vi "AWG Set and Arm.vi"(8 "error in (no error)":errorcluster, 10 "T [s] (1ms)":dbl=0.001, 11 "awg session in":T1) -> (0 "error out":errorcluster, 3 "awg session out":T1)   [LabVIEW 2018, in "AWG.lvlib"]
doc: "AWG wrapper: This sets the AWG to desired frequency and arms it. No pulses are generated here. Waiting for trigger!"
uses:
  AWG.lvlib
  AWG Session.ctl
  AWG Type.ctl
  Agilent 33XXX Series/Agilent 33XXX Series.lvlib
  AFG3000/Tektronix AFG 3000 Series.lvlib
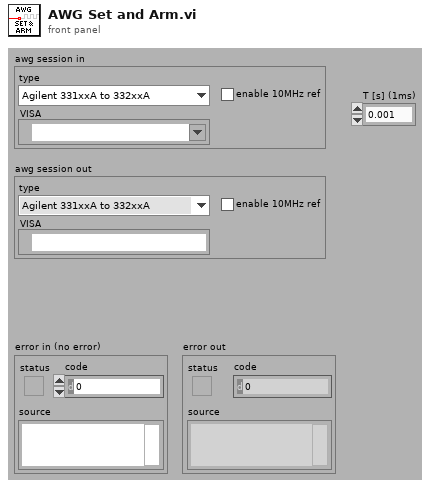
[diagram p1: front panel]
types:
  T1 = typedef "AWG.lvlib/AWG Session.ctl" = cluster{"type":T2, "VISA":refnum<visa-resource-name>, "enable 10MHz ref":bool}
  T2 = typedef "AWG.lvlib/AWG Type.ctl" = enum16{"Agilent 331xxA to 332xxA", "Agilent 335xxA to 336xxA", "Tektronix AFG3101C", "dummy"}
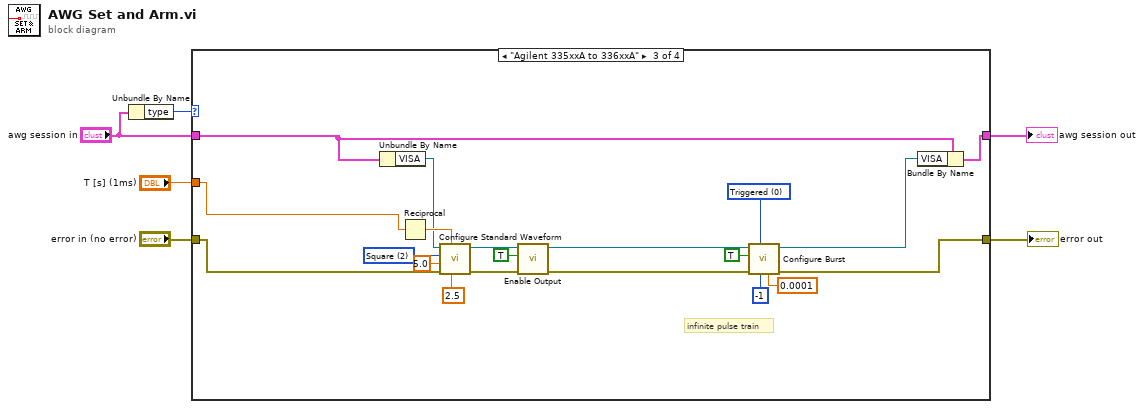
[diagram p0: block diagram]
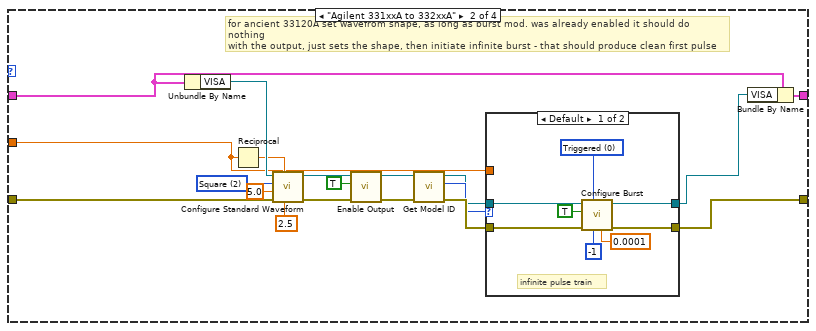
[diagram p3: hidden frame]
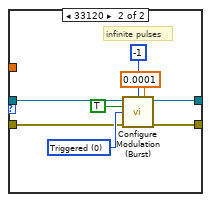
[diagram p4: hidden frame]
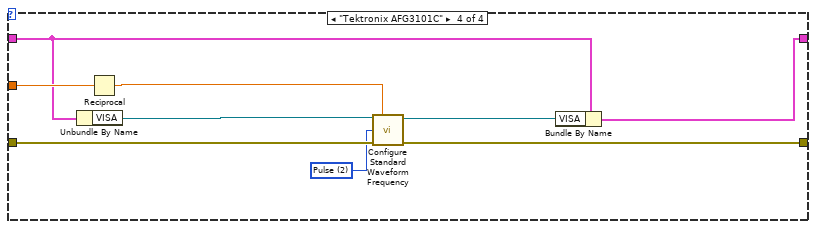
[diagram p5: hidden frame]
diagram:
  n1 = Unbundle By Name("awg session in") -> ("type"=w6:T2)
  n2 = case shown="\"Agilent 335xxA to 336xxA\"" w6 {
    tunnel: "error in (no error)" -> [w8 w22 w52 w67]
    tunnel: [w8 w10 w45 w64] -> w4
    tunnel: "awg session in" -> [w7 w26 w63 w71]
    tunnel: [w7 w27 w62 w70] -> w2
    tunnel: "T [s] (1ms)" -> [_ w11 w53 w72]
    frame Default {
    }
    frame "Agilent 331xxA to 332xxA" {
      w25 = u16 2 items=["DC", "Sine", "Square", "Triangle", "Ramp", "Pulse", "Noise", "Sinc", "Negative Ramp", "Exponential Rise", "Exponential Fall", "Cardiac"] ("Waveform Function (1: Sine)")
      # "for ancient 33120A set wavefrom shape, as long as burst mod. was already enabled it should do nothing\nwith the output, just sets the shape, then initiate infinite burst - that should produce clean first pulse"
      n3 = Unbundle By Name(w26) -> ("VISA"=w23:refnum<visa-resource-name>)
      n4 = Reciprocal(x=w11) -> (1/x=w12:dbl)
      n5 = call "Configure Standard Waveform.vi"("DC Offset (0.00 V)"=2.5, "Frequency (1000 Hz)"=w12, "error in (no error)"=w22, "Amplitude (1)"=5.0, "Waveform Function (1: Sine)"=w25, "VISA resource name"=w23) -> ("error out"=w20:errorcluster, "VISA resource name out"=w19:refnum<visa-resource-name>)  [unwired: 4 in]
      n6 = call "Enable Output.vi"("error in (no error)"=w20, "Enable Output  (T: Enable)"=TRUE, "VISA resource name"=w19) -> ("error out"=w17:errorcluster, "VISA resource name out"=w16:refnum<visa-resource-name>)  [unwired: 7 in]
      n7 = call "Get Model ID.vi"("error in (no error)"=w17, "VISA resource name"=w16) -> ("error out"=w15:errorcluster, "model ID"=w14:u32, "VISA resource name out"=w13:refnum<visa-resource-name>)  [unwired: 7 in]
      n8 = case shown="Default" w14 {
        tunnel: [w34 w40] -> w10
        tunnel: [w33 w39] -> w9
        tunnel: w11 -> [_ _]
        tunnel: w15 -> [w35 w38]
        tunnel: w13 -> [w32 w37]
        frame Default {
          w31 = u16 0 items=["Triggered", "Gated"] ("Burst Mode (0: Triggered)")
          # "infinite pulse train"
          n9 = call "Configure Burst.vi"("Burst Period (1 s)"=0.0001, "Burst Count (1)"=-1, "Burst Mode (0: Triggered)"=w31, "error in (no error)"=w35, "Enable Burst (T: Enable)"=TRUE, "VISA resource name"=w32) -> ("error out"=w34:errorcluster, "VISA resource name out"=w33:refnum<visa-resource-name>)  [unwired: 4 in]
        }
        frame 33120 {
          w41 = u16 0 items=["Triggered", "Gated"] ("Burst Modulation Mode (0: Triggered)")
          # "infinite pulses"
          n10 = call "Configure Modulation (Burst).vi"("VISA resource name"=w37, "Burst Count (1)"=-1, "Burst Period (1 s)"=0.0001, "Enable Burst Modulation (T: Enable)"=TRUE, "Burst Modulation Mode (0: Triggered)"=w41, "error in (no error)"=w38) -> ("VISA resource name out"=w39:refnum<visa-resource-name>, "error out"=w40:errorcluster)  [unwired: 8 in]
        }
      }
      n11 = Bundle By Name(cluster=w26, "VISA"=w9) -> (w27:T1)
    }
    frame "Agilent 335xxA to 336xxA" {
      w51 = u16 0 items=["Triggered", "Gated"] ("Burst Mode (0: Triggered)")
      w61 = u16 2 items=["DC", "Sine", "Square", "Triangle", "Ramp", "Pulse", "Noise", "Sinc", "Negative Ramp", "Exponential Rise", "Exponential Fall", "Cardiac"] ("Waveform Function (1: Sine)")
      # "infinite pulse train"
      n12 = Unbundle By Name(w63) -> ("VISA"=w54:refnum<visa-resource-name>)
      n13 = Reciprocal(x=w53) -> (1/x=w55:dbl)
      n14 = call "Configure Standard Waveform.vi"("DC Offset (0.00 V)"=2.5, "Frequency (1000 Hz)"=w55, "error in (no error)"=w52, "Amplitude (1)"=5.0, "Waveform Function (1: Sine)"=w61, "VISA resource name"=w54) -> ("error out"=w58:errorcluster, "VISA resource name out"=w57:refnum<visa-resource-name>)  [unwired: 4 in]
      n15 = call "Enable Output.vi"("error in (no error)"=w58, "Enable Output  (T: Enable)"=TRUE, "VISA resource name"=w57) -> ("error out"=w47:errorcluster, "VISA resource name out"=w46:refnum<visa-resource-name>)  [unwired: 7 in]
      n16 = call "Configure Burst.vi"("Burst Period (1 s)"=0.0001, "Burst Count (1)"=-1, "Burst Mode (0: Triggered)"=w51, "error in (no error)"=w47, "Enable Burst (T: Enable)"=TRUE, "VISA resource name"=w46) -> ("error out"=w45:errorcluster, "VISA resource name out"=w44:refnum<visa-resource-name>)  [unwired: 4 in]
      n17 = Bundle By Name(cluster=w63, "VISA"=w44) -> (w62:T1)
    }
    frame "Tektronix AFG3101C" {
      w66 = u16 2 items=["Sine", "Square", "Pulse", "Ramp", "Noise", "DC", "Sin(x)/x", "Gaussian", "Lorentz", "Exponential Rise", "Exponential Decay", "Haversine"] ("Waveform Function (0: Sine)")
      n18 = Unbundle By Name(w71) -> ("VISA"=w68:refnum<visa-resource-name>)
      n19 = Reciprocal(x=w72) -> (1/x=w69:dbl)
      n20 = call "Configure Standard Waveform Frequency.vi"("VISA resource name"=w68, "Frequency (1000 Hz)"=w69, "Waveform Function (0: Sine)"=w66, "error in (no error)"=w67) -> ("VISA resource name out"=w65:refnum<visa-resource-name>, "error out"=w64:errorcluster)  [unwired: 10 in]
      n21 = Bundle By Name(cluster=w71, "VISA"=w65) -> (w70:T1)
    }
  }
  "error out" <- w4
  "awg session out" <- w2
